vi "new_inline_table.vi"(8 "error in (no error)":errorcluster) -> (0 "error out":errorcluster, 3 "InlineTable out":refnum<class "InlineTable.lvclass">)   [LabVIEW 2020, in "toml_edit.lvlib" / "InlineTable.lvclass"]
uses:
  InlineTable.lvclass
  InlineTable.lvclass/InlineTable.ctl
  dragon_toml_64.dll
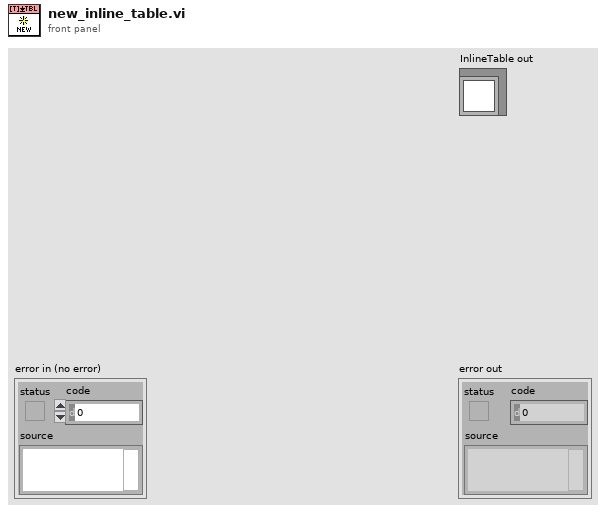
[diagram p1: front panel]
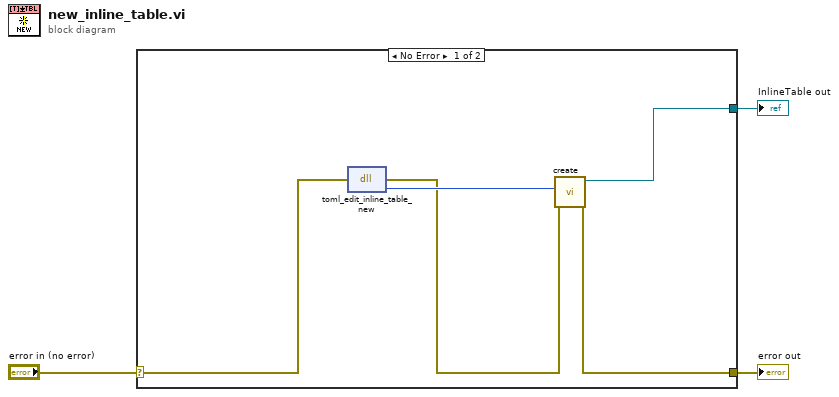
[diagram p0: block diagram]
diagram:
  n1 = case shown="No Error" "error in (no error)" {
    selector: "error in (no error)" -> [w6 w9]
    tunnel: [w4 w9] -> w2
    tunnel: [w8 _] -> w1
    frame No Error {
      n2 = dll-call lib="C:/Projects/labview-project-load-tools/source/submodules/toml-edit-labview/lv_src/dragon_toml_*.*" fn="toml_edit_inline_table_new"(error in=w6) -> (error out=w5:errorcluster, "inline_table_ref"=w7:u64)  [unwired: 2 in, 1 out]
      n3 = call "create.vi"("error in (no error)"=w5, "ref"=w7) -> ("error out"=w4:errorcluster, "InlineTable out"=w8:refnum<class "InlineTable.lvclass">)  [unwired: 8 in]
    }
    frame Error {
    }
  }
  "error out" <- w2
  "InlineTable out" <- w1
